vi "Set_Source_Data.vi"(8 "error in (no error)":errorcluster, 10 "data":T1, 11 "Class in":refnum<class "AB_Source.lvclass">) -> (0 "error out":errorcluster, 3 "Class out":refnum<class "AB_Source.lvclass">)   [LabVIEW 2020, in "AB_Source.lvclass"]
uses:
  <vilib>/AppBuilder/AB_Classes/Source/AB_Source.lvclass
  <vilib>/AppBuilder/AB_Classes/Source/AB_Source.ctl
  <vilib>/AppBuilder/AB_Source_Inclusion.ctl
  <vilib>/AppBuilder/AB_Source_Properties.ctl
  <vilib>/AppBuilder/AB_Source_Property_Type.ctl
  <vilib>/AppBuilder/AB_Classes/Source/AB_Source.lvclass/AB_Source.ctl
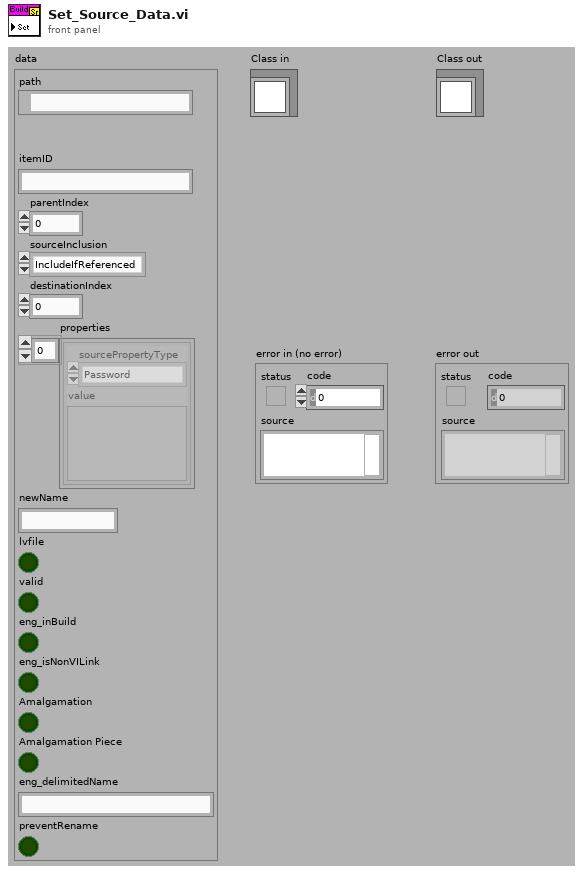
[diagram p1: front panel]
types:
  T1 = typedef "AB_Source.ctl" = cluster{"path":path, "itemID":string, "parentIndex":i32, "sourceInclusion":T2, "destinationIndex":i32, "properties":T3[], "newName":string, "lvfile":bool, "valid":bool, "eng_inBuild":bool, "eng_isNonVILink":bool, "Amalgamation":bool, "Amalgamation Piece":bool, "eng_delimitedName":string, "preventRename":bool}
  T2 = typedef "AB_Source_Inclusion.ctl" = enum16{"IncludeIfReferenced", "Include", "Exclude", "TopLevel"}
  T3 = typedef "AB_Source_Properties.ctl" = cluster{"sourcePropertyType":T4, "value":variant}
  T4 = typedef "AB_Source_Property_Type.ctl" = enum16{"Remove block diagram", "Remove front panel", "Password", "Window has title bar", "Show menu bar", "Show vertical scroll bar", "Show horizontal scroll bar", "Show toolbar", "Show Abort button", "Show fp when called", "Window behavior", "Allow user to close window", "Window run-time position", "Run when opened", "Allow debugging", "Auto error handling", "Generate guard code", "Use stack variables", "Expression folding", "Integer only", "Inline subVI"}
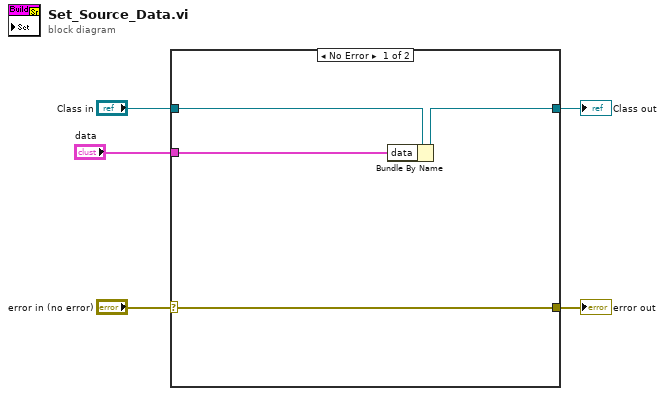
[diagram p0: block diagram]
diagram:
  n1 = case "Case" shown="No Error" "error in (no error)" {
    selector: "error in (no error)" -> [w9 w11]
    tunnel: [w9 w11] -> w4
    tunnel: [w8 w10] -> w2
    tunnel: "Class in" -> [w7 w10]
    tunnel: "data" -> [w6 _]
    frame No Error {
      n2 = Bundle By Name(cluster=w7, "data"=w6) -> (w8:refnum<class "AB_Source.lvclass">)
    }
    frame Error {
    }
  }
  "error out" <- w4
  "Class out" <- w2
